vi "Add To Log.vi"(10 "Debug Data in":refnum<class "Debug Data.lvclass">, 11 "Debug Log in":refnum<class "Debug Log.lvclass">) -> (2 "Debug Data Out":refnum<class "Debug Data.lvclass">, 3 "Debug Log out":refnum<class "Debug Log.lvclass">)   [LabVIEW 2020, in "Debug Log.lvclass"]
uses:
  Debug Log.lvclass
  Debug Data/Debug Data.lvclass
  Debug Data/Debug Data.lvclass/Debug Data.ctl
  Debug Log.lvclass/Debug Log.ctl
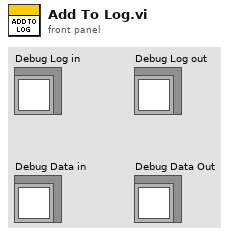
[diagram p1: front panel]
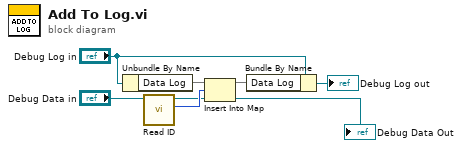
[diagram p0: block diagram]
diagram:
  n1 = Unbundle By Name("Debug Log in") -> ("Data Log"=w7:map{u32, refnum<class "Debug Data.lvclass">})
  n2 = call "Read ID.vi"("Debug Data in"="Debug Data in") -> ("ID"=w5:u32, "Debug Data out"=w4:refnum<class "Debug Data.lvclass">)  [unwired: 9 in]
  n3 = Insert Into Map(map in=w7, key=w5, value=w4) -> (map out=w2:map{u32, refnum<class "Debug Data.lvclass">})  [unwired: 2 out]
  n4 = Bundle By Name(cluster="Debug Log in", "Data Log"=w2) -> (→"Debug Log out":refnum<class "Debug Log.lvclass">)
  "Debug Data Out" <- "Debug Data in"
